vi "Add VI to Library.vi"(6 "Library Folder":string, 7 "Current Bus Path":path=path "D:/Documents/Projects/SPIAPI/IOEngineCode/Initialize Node Resources.vi", 8 "error in":errorcluster, 9 "Bus Number":i32, 10 "VI Name":string, 11 "Path to new VI":path) -> (0 "error out":errorcluster, 3 "Path to new IO Node":path)   [LabVIEW 2014, in "SPI Engine Scripting.lvlib"]
uses:
  SPI Engine Scripting.lvlib
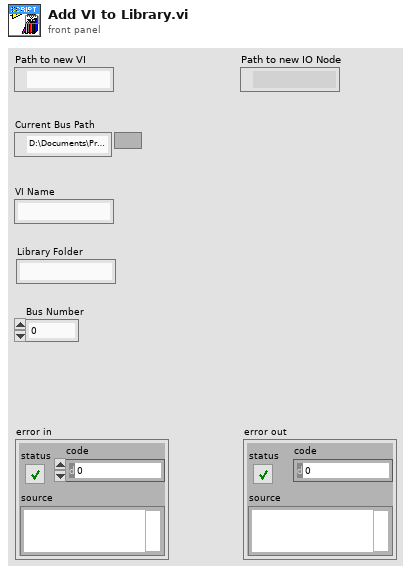
[diagram p1: front panel]
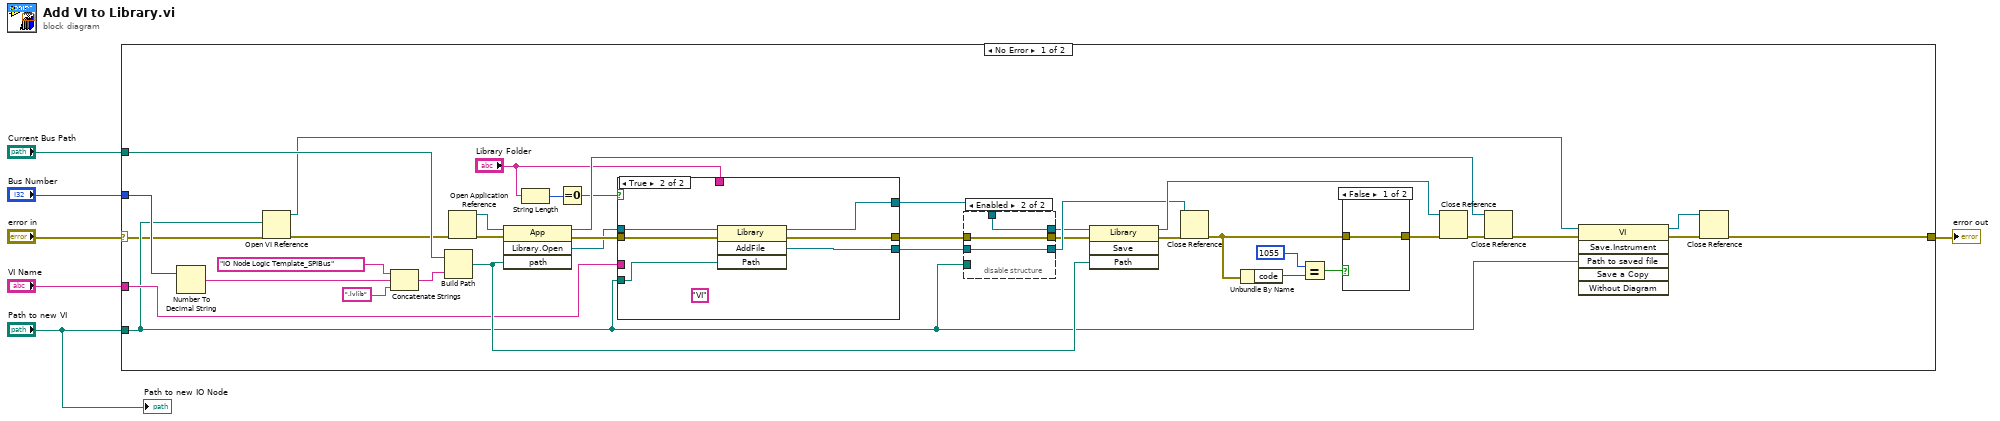
[diagram p0: block diagram]
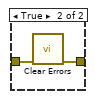
[diagram p2: hidden frame]
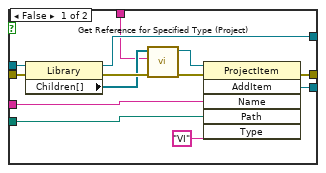
[diagram p3: hidden frame]
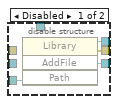
[diagram p4: hidden frame]
diagram:
  n1 = case shown="No Error" "error in" {
    selector: "error in" -> [w8 w74]
    tunnel: "VI Name" -> [w24 _]
    tunnel: [w11 w74] -> w4
    tunnel: "Path to new VI" -> [w10 _]
    tunnel: "Current Bus Path" -> [w33 _]
    tunnel: "Bus Number" -> [w23 _]
    frame No Error {
      n2 = Number To Decimal String(number=w23) -> (decimal integer string=w32:string)  [unwired: 1 in]
      n3 = Open VI Reference(vi path=w10, error in (no error)=w8) -> (vi reference=w14:refnum<vi>, error out=w7:errorcluster)  [unwired: 4 in]
      n4 = Concatenate Strings("IO Node Logic Template_SPIBus" ("name or relative path"), w32, ".lvlib" ("string")) -> (w41:string)
      n5 = Build Path(base path=w33, name or relative path=w41) -> (appended path=w38:path)
      n6 = Open Application Reference(8:w7) -> (0:w42:errorcluster, 3:w43:refnum<vi>)  [unwired: 3 in]
      n7 = invoke class="App" method="Library.Open"(reference=w43, error in=w42, "path"=w38) -> (reference out=w28:refnum<vi>, error out=w31:errorcluster, "Open Library"=w30:refnum<vi>)  [unwired: 1 in, 1 out]
      n8 = String Length(string="Library Folder") -> (length=w21:i32)
      n9 = Equal To 0?(x=w21) -> (x = 0?=w20:bool)
      n10 = case shown="True" w20 {
        tunnel: w31 -> [w60 w65]
        tunnel: w30 -> [w59 w66]
        tunnel: [w54 w64] -> w27
        tunnel: [w53 w63] -> w26
        tunnel: [w52 w62] -> w25
        tunnel: w10 -> [w51 w61]
        tunnel: w24 -> [w49 _]
        tunnel: "Library Folder" -> [w48 _]
        frame False {
          n11 = property class="Library"(reference=w59, error in=w60) -> (reference out=w54:refnum<vi>, error out=w58:errorcluster, "Children[]"=w55:refnum<vi>[])
          n12 = call "Get Reference for Specified Type (Project).vi"("error in (no error)"=w58, "Type to Find"=w48, "Array of References"=w55) -> ("error out"=w57:errorcluster, "Project Item"=w56:refnum<vi>)  [unwired: 6 in, 1 out]
          n13 = invoke class="ProjectItem" method="AddItem"(reference=w56, error in=w57, "Name"=w49, "Path"=w51, "Type"="VI") -> (error out=w53:errorcluster, "AddItem"=w52:refnum<vi>)  [unwired: 1 in, 4 out]
        }
        frame True {
          (unwired) "VI" ("Type")
          n14 = invoke class="Library" method="AddFile"(reference=w66, error in=w65, "Path"=w61) -> (reference out=w64:refnum<vi>, error out=w63:errorcluster, "AddFile"=w62:refnum<vi>)  [unwired: 1 in, 1 out]
        }
      }
      n15 = disable-structure shown="Enabled" {
        disable-tunnel: [w70 w71] -> w37
        disable-tunnel: [w69 w72] -> w36
        disable-tunnel: [w68 w73] -> w35
        disable-tunnel: w10 -> [w67 _]
        disable-tunnel: w27 -> [_ w73]
        disable-tunnel: w26 -> [_ w72]
        disable-tunnel: w25 -> [_ w71]
        frame Disabled {
          n16 = invoke class="Library" method="AddFile"("Path"=w67) -> (reference out=w68:refnum<vi>, error out=w69:errorcluster, "AddFile"=w70:refnum<vi>)  [unwired: 3 in, 1 out]
        }
        frame Enabled {
        }
      }
      n17 = invoke class="Library" method="Save"(reference=w35, error in=w36, "Path"=w38) -> (reference out=w40:refnum<vi>, error out=w39:errorcluster)  [unwired: 1 in, 2 out]
      n18 = Close Reference(reference=w37, error in (no error)=w39) -> (error out=w16:errorcluster)
      n19 = Unbundle By Name(w16) -> ("code"=w17:i32)
      n20 = Equal?(x=1055, y=w17) -> (x = y?=w18:bool)
      n21 = case shown="False" w18 {
        tunnel: w16 -> [w45 w47]
        tunnel: [w45 w46] -> w15
        frame False {
        }
        frame True {
          n22 = call <vilib>:"Clear Errors.vi"("error in (no error)"=w47) -> ("error out"=w46:errorcluster)  [unwired: 5 in, 1 out]
        }
      }
      n23 = Close Reference(reference=w40, error in (no error)=w15) -> (error out=w29:errorcluster)
      n24 = Close Reference(reference=w28, error in (no error)=w29) -> (error out=w9:errorcluster)
      n25 = invoke class="VI" method="Save.Instrument"(reference=w14, error in=w9, "Path to saved file"=w10) -> (reference out=w12:refnum<vi>, error out=w13:errorcluster)  [unwired: 3 in, 4 out]
      n26 = Close Reference(reference=w12, error in (no error)=w13) -> (error out=w11:errorcluster)
    }
    frame Error {
    }
  }
  "error out" <- w4
  "Path to new IO Node" <- "Path to new VI"
